vi "AlliGator Update Phasor Image Elements to Update.vi"(8 "Error In":errorcluster, 9 "CtlRef":refnum<vi>, 11 "Phasor Plot Element to Update":string) -> (0 "Error Out":errorcluster, 3 "Phasor Plot Image Elements to Update":string[](array[string]))   [LabVIEW 2021, in "AlliGator Phasor Plot.lvlib"]
doc: "Modifies the list of Phasor Plot image elements to update based on user selection."
uses:
  AlliGator Phasor Plot.lvlib
  AlliGator Variables List.ctl
  AlliGator Globals, Variables & Constants.lvlib
  Strings/Strings.lvlib
panel:
  # "see the AlliGator License on the block diagram (Ctrl+E or Window:Show Block Diagram)"
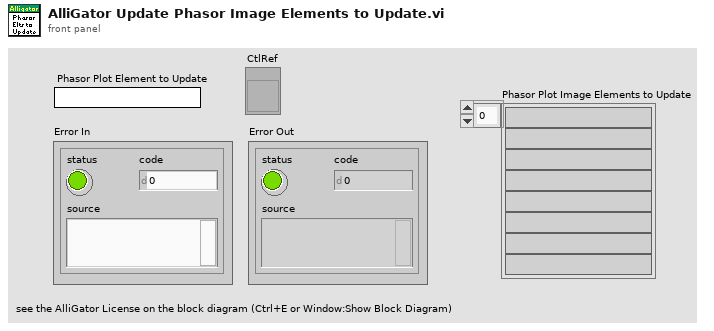
[diagram p1: front panel]
types:
  T1 = typedef "AlliGator Globals, Variables & Constants.lvlib/AlliGator Variables List.ctl" = enum16{"---- GUI ----", "Initialization Status", "State Indicators Refnum", "Original AlliGator Menu Items", "Current Action Loop State", "Script in progress", "Playback", "Loop Playback", "Search ROI Used", "Search ROI", "Decay Graph Max Legend Size", "Intensity Graph Max Legend Size", "Decay Statistics Graph Max Legend Size", "Phasor Graph Max Legend Size", "Phasor Ratio Graph Max Legend Size", "Lifetime Graph Max Legend Size", "---- Files ----", "Export Dataset Frames as Individual Files", "Show Batch Export Help Balloons", "Frames in Dataset", "ptu File Frame Start Indices", "Current Frame in Dataset", "Current Frame Timestamp", "------ Python Plugins ------", "Python Plugins Information", "Python Session", "Valid Python Session?", "---- Source Image ----", "Dataset Loaded", "Dataset Metadata", "Dataset Channel", "Dataset Data Description", "Background Dataset Metadata", "Background Dataset Channel", "Background Dataset Data Description", "Background File Subtraction", "Background File Path", "Background File Pile-up Correction", "Background File Pixel Well Capacity", "Background File Scaling Factor", "Source Image ROIs", "Current Source Image ROI", "Source Image ROI Event Refnum", "X_Source Image Display Range", "X_Source Image Palette Information", "Source Image Palette List", "Source Image Scale", "Current Dataset Load Settings", "Source Image:ROI Overlay Color", "---- Image Profile Window ----", "Image Profile:Overlay ROI in Source Image", "Image Profile Window Event Refnum", "Image Profile:IntensityType", "Image Profile:Intensity Average Type", "Image Profile:Intensity-weighted SDV", "Image Profile:Box Profile Type", "Image Profile Window Open", "Image Profile:Plotted Fit Parameter", "X_Type of Displayed Image", "X_Time Gate Slider", "Dataset Path", "Source Image Overlay to Erase", "Is Displayed Image Accumulated", "White Light Image Modified", "Mask Image Modified", "Macrotime Gate Separation", "------ Phasor Graph -------", "Phasor Graph:Show Line", "---- Phasor Plot ---", "Phasor Plot Parameters Changed", "FLI Dataset Modified since last Phasor Plot Calculation", "Phasor Harmonics Data", "Selected Phasor Harmonics", "Phasor Harmonic Manager Event Refnum", "Phasor Plot ROIs", "Current Phasor Plot ROI", "Phasor Plot ROI Event Refnum", "Phasor Plot Image Reference Points", "Phasor Plot Computed", "Phasor Plot Palette Information", "Phasor Plot Palette List", "Phasor Ratio Palette Information", "Phasor Ratio Palette List", "Phasor Image Scale", "Phasor Plot Image Overlay to Erase", "Phasor Plot Image Elements to Update", "Current Phasor Plot Calculation Parameters", "Current Phasor Calibration Options", "Reset Cumulated Phasor Plot", "Phasor Ratio Reference 1", "Phasor Ratio Lifetime Reference 1", "Phasor Ratio Reference 1 Frequency", "Phasor Ratio Reference 2", "Phasor Ratio Lifetime Reference 2", "Phasor Ratio Reference 2 Frequency", "---- Decay Analysis ----", "Number of Selected Decays to Fit", "LS Fit Results", "LAR Fit Results", "BS Fit Results", "Last Decay Max - Min", "Best Fit Parameters", "Best Fit Parameter Names", "Actual Size X", "Actual Size Y", "Binning X", "Binning Y", "Actual # Gates", "Dataset Number", "Gates to...", "Gates Skipped", "Gates to keep", "Gate Step", "Gate Separation", "Reversed Gates", "Pile-up Correction", "Pixel Well Capacity", "Background Subtracted", "Background Subtraction Method", "Background Definition Range", "Background File (deprecated)", "Number of Dataset Accumulated", "Array of Accumulated Dataset Paths", "Do Averaged Datasets", "Destination File Path", "Process Plot Target", "Use 1/D as Phasor Frequency", "---- Decay Fit Parameter Map -----", "Decay Fit Parameter Map Palette Information", "Decay Fit Parameter Map Palette List", "Local Decay Graph Window Event Refnum", "------- Local Decay Window ---------", "Use normalized IRF for convolution", "----- Miscellaneous ----", "Skippable Dialog Windows Status"}
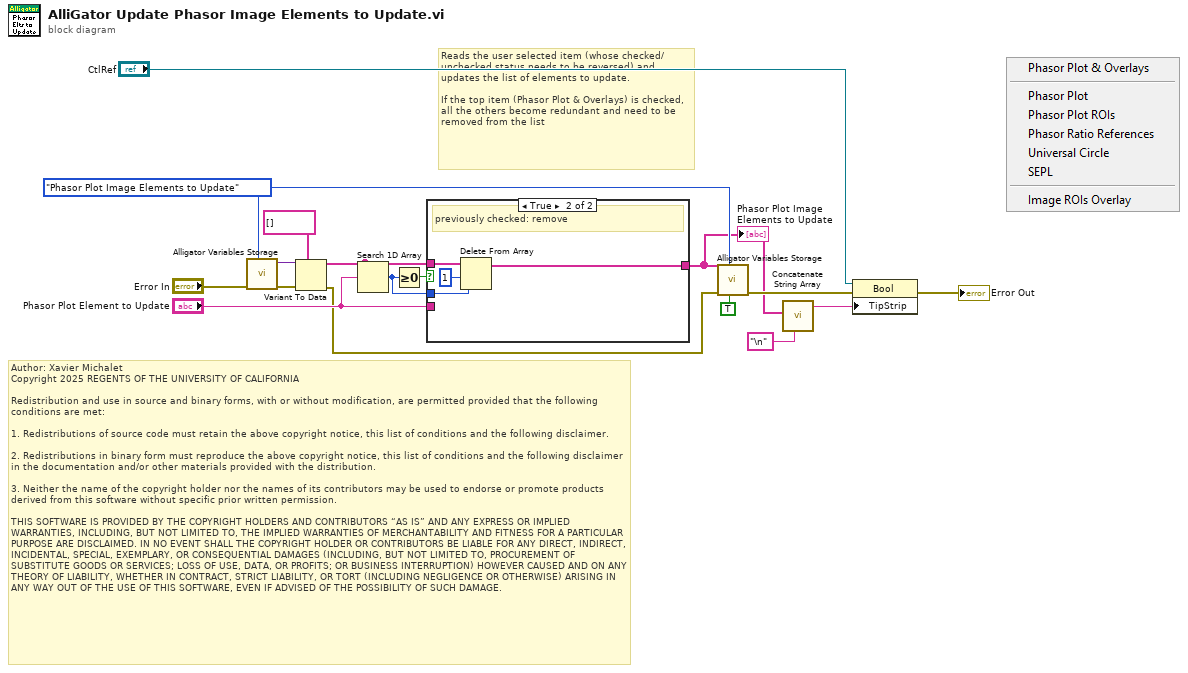
[diagram p0: block diagram]
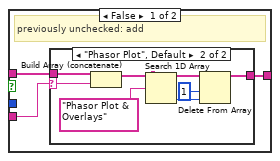
[diagram p2: hidden frame]
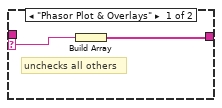
[diagram p3: hidden frame]
diagram:
  w9 = AlliGator_Variables_List."Phasor Plot Image Elements to Update" ("Alligator Variable")
  # "Author: Xavier Michalet\nCopyright 2025 REGENTS OF THE UNIVERSITY OF CALIFORNIA\n\nRedistribution and use in source and binary forms, with or without modification, are permitted provided that the following conditions are met:\n\n1. Redistributions of source code must retain the above copyright notice, this list of conditions and the following disclaimer.\n\n2. Redistributions in binary form must reproduce the above copyright notice, this list of conditions and the following disclaimer in the documentation and/or other materials provided with the distribution.\n\n3. Neither the name of the copyright holder nor the names of its contributors may be used to endorse or promote products derived from this software without specific prior written permission.\n\nTHIS SOFTWARE IS PROVIDED BY THE COPYRIGHT HOLDERS AND CONTRIBUTORS “AS IS” AND ANY EXPRESS OR IMPLIED WARRANTIES, INCLUDING, BUT NOT LIMITED TO, THE IMPLIED WARRANTIES OF MERCHANTABILITY AND FITNESS FOR A PARTICULAR PURPOSE ARE DISCLAIMED. IN NO EVENT SHALL THE COPYRIGHT HOLDER OR CONTRIBUTORS BE LIABLE FOR ANY DIRECT, INDIRECT, INCIDENTAL, SPECIAL, EXEMPLARY, OR CONSEQUENTIAL DAMAGES (INCLUDING, BUT NOT LIMITED TO, PROCUREMENT OF SUBSTITUTE GOODS OR SERVICES; LOSS OF USE, DATA, OR PROFITS; OR BUSINESS INTERRUPTION) HOWEVER CAUSED AND ON ANY THEORY OF LIABILITY, WHETHER IN CONTRACT, STRICT LIABILITY, OR TORT (INCLUDING NEGLIGENCE OR OTHERWISE) ARISING IN ANY WAY OUT OF THE USE OF THIS SOFTWARE, EVEN IF ADVISED OF THE POSSIBILITY OF SUCH DAMAGE."
  # "Reads the user selected item (whose checked/unchecked status needs to be reversed) and updates the list of elements to update.\n\nIf the top item (Phasor Plot & Overlays) is checked, all the others become redundant and need to be removed from the list"
  n1 = call "Alligator Variables Storage.vi"("AlliGator Variable"=w9, "Error In"="Error In") -> ("Error Out"=w16:errorcluster, "Data out"=w17:variant)  [unwired: 7 in, 1 out]
  n2 = Variant To Data(error in=w16, type=string[] [], Variant=w17) -> (data=w11:string[], error out=w8:errorcluster)
  n3 = Search 1D Array(1D array=w11, element="Phasor Plot Element to Update") -> (index of element=w12:i32)  [unwired: 1 in]
  n4 = Greater Or Equal To 0?(x=w12) -> (x >= 0?=w13:bool)
  n5 = case shown="True" w13 {
    tunnel: w12 -> [_ w32]
    tunnel: w11 -> [w20 w33]
    tunnel: [w18 w30] -> w2
    tunnel: "Phasor Plot Element to Update" -> [w19 _]
    frame False {
      # "previously unchecked: add"
      n6 = case shown="\"Phasor Plot\", Default" w19 {
        selector: w19 -> [w22 w28]
        tunnel: w20 -> [_ w29]
        tunnel: [w21 w24] -> w18
        frame "Phasor Plot & Overlays" {
          # "unchecks all others"
          n7 = Build Array(w22) -> (w21:string[])
        }
        frame "Phasor Plot", Default {
          n8 = Build Array (concatenate)(w29, w28) -> (w26:string[])
          n9 = Search 1D Array(1D array=w26, element="Phasor Plot & Overlays") -> (index of element=w25:i32)  [unwired: 1 in]
          n10 = Delete From Array(array=w26, length=1, index=w25) -> (array with subset deleted=w24:string[])  [unwired: 1 out]
        }
      }
    }
    frame True {
      # "previously checked: remove"
      n11 = Delete From Array(array=w33, length=1, index=w32) -> (array with subset deleted=w30:string[])  [unwired: 1 out]
    }
  }
  "Phasor Plot Image Elements to Update" <- w2
  n12 = call "Alligator Variables Storage.vi"("Get(F)/Set"=TRUE, "AlliGator Variable"=w9, "Error In"=w8, "Data in"=w2) -> ("Error Out"=w5:errorcluster)  [unwired: 5 in, 2 out]
  n13 = call "Concatenate String Array.vi"("Separator (TAB)"="\n", "String Array"=w2) -> ("Formatted String"=w3:string)  [unwired: 9 in]
  n14 = property class="Bool"(reference="CtlRef", error in=w5, "TipStrip"=w3) -> (error out=→"Error Out":errorcluster)  [unwired: 1 out]
